vi "image calibrating and processing.vi"(3 "error in":errorcluster) -> (0 "error out":errorcluster, 1 "Objects Array":cluster{"X Coord":dbl[], "Y Coord":dbl[]}[](array[cluster]), 2 "Image Out (duplicate)":T1)   [LabVIEW 2009]
uses:
  <vilib>/vision/NI_Vision_Development_Module.lvlib
  <vilib>/vision/Image Controls.llb/IMAQ Image.ctl
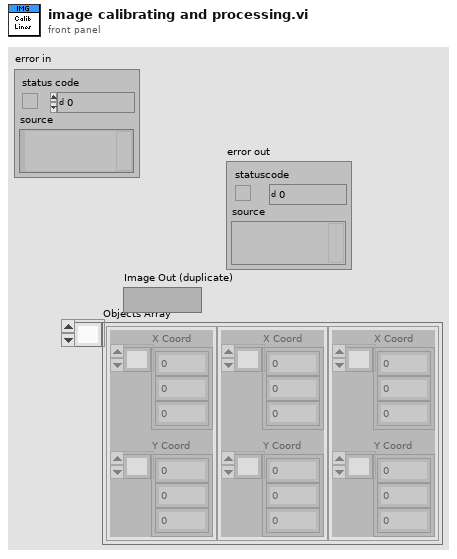
[diagram p1: front panel]
types:
  T1 = typedef "IMAQ Image.ctl" = refnum<image>
  T2 = enum32{"AutoM", "Close", "Dilate", "Erode", "Gradient", "Gradient out", "Gradient in", "Hit miss", "Open", "PClose", "POpen", "Thick", "Thin"}
  T3 = cluster{"Measurement Parameter":i32, "Range Lower Value":dbl, "Range Upper Value":dbl, "Range":bool, "Measurement Type":bool}[]
  T4 = typedef "Image Type" = u32
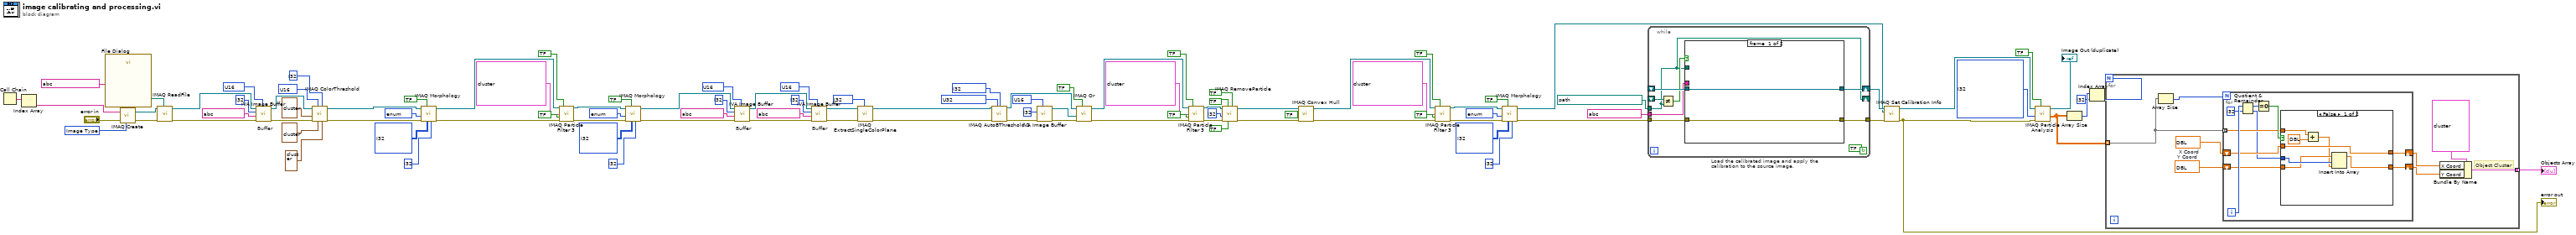
[diagram p0: block diagram]
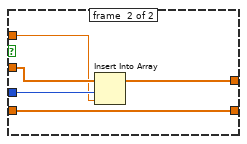
[diagram p2: hidden frame]
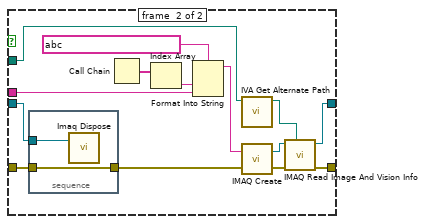
[diagram p3: hidden frame]
diagram:
  w10 = i32[] ? items=["Center of Mass X", "Center of Mass Y", "First Pixel X", "First Pixel Y", "Bounding Rect Left", "Bounding Rect Top", "Bounding Rect Right", "Bounding Rect Bottom", "Max Feret Diameter Start X", "Max Feret Diameter Start Y", "Max Feret Diameter End X", "Max Feret Diameter End Y", "Max Horiz. Segment Length Left", "Max Horiz. Segment Length Right", "Max Horiz. Segment Length Row", "-", "Bounding Rect Width", "Bounding Rect Height", "Bounding Rect Diagonal", "Perimeter", "Convex Hull Perimeter", "Holes' Perimeter", "Max Feret Diameter", "Equivalent Ellipse Major Axis", "Equivalent Ellipse Minor Axis", "Equivalent Ellipse Minor Axis (Feret)", "Equivalent Rect Long Side", "Equivalent Rect Short Side", "Equivalent Rect Diagonal", "Equivalent Rect Short Side (Feret)", "Average Horiz. Segment Length", "Average Vert. Segment Length", "Hydraulic Radius", "Waddel Disk Diameter", "-", "Area", "Holes' Area", "Particle & Holes' Area", "Convex Hull Area", "Image Area", "-", "Number of Holes", "Number of Horiz. Segments", "Number of Vert. Segments", "-", "Orientation", "Max Feret Diameter Orientation", "-", "% Area/Image Area", "% Area/(Particle & Holes' Area)", "Ratio of Equivalent Ellipse Axes", "Ratio of Equivalent Rect Sides", "-", "Elongation Factor", "Compactness Factor", "Heywood Circularity Factor", "Type Factor", "-", "Sum X", "Sum Y", "Sum XX", "Sum XY", "Sum YY", "Sum XXX", "Sum XXY", "Sum XYY", "Sum YYY", "-", "Moment of Inertia XX", "Moment of Inertia XY", "Moment of Inertia YY", "Moment of Inertia XXX", "Moment of Inertia XXY", "Moment of Inertia XYY", "Moment of Inertia YYY", "Norm. Moment of Inertia XX", "Norm. Moment of Inertia XY", "Norm. Moment of Inertia YY", "Norm. Moment of Inertia XXX", "Norm. Moment of Inertia XXY", "Norm. Moment of Inertia XYY", "Norm. Moment of Inertia YYY", "Hu Moment 1", "Hu Moment 2", "Hu Moment 3", "Hu Moment 4", "Hu Moment 5", "Hu Moment 6", "Hu Moment 7"] ("Real-World Measurements")
  w46 = u16 ? items=["Push", "Pop", "Reset"] ("Function")
  w48 = i32 ? items=["clustering", "entropy", "metric", "moments", "inter-class variance"] ("Method")
  w49 = u32 ? items=["Bright Objects", "Dark Objects"] ("Look For")
  w54 = i32 ? items=["Red", "Green", "Blue", "Hue", "Saturation", "Luminance", "Value", "Intensity"] ("Color Plane")
  w57 = u16 ? items=["Push", "Pop", "Reset"] ("Function")
  w62 = u16 ? items=["Push", "Pop", "Reset"] ("Function")
  w87 = u16 ? items=["RGB", "HSL", "HSV", "HSI"] ("Color Mode")
  w91 = u16 ? items=["Push", "Pop", "Reset"] ("Function")
  w94 = T4 ? items=["Grayscale (U8)", "Grayscale (I16)", "Grayscale (SGL)", "Complex (CSG)", "RGB (U32)", "HSL (U32)", "RGB (U64)", "Grayscale (U16)"] ("Image Type")
  # "Buffer"
  # "Buffer"
  # "Buffer"
  n1 = Call Chain() -> (call chain=w98:string[])
  n2 = Index Array(array=w98) -> (element=w97:string)  [unwired: 1 in]
  n3 = call "File Dialog"("prompt"=string ?) -> ("selected path"=w95:path)  [unwired: 6 in, 8 out]
  n4 = call "IMAQ Create"("Image Name"=w97, "Image Type"=w94, "error in (no error)"="error in") -> ("New Image"=w101:T1, "error out"=w100:errorcluster)  [unwired: 1 in, 1 out]
  n5 = call "IMAQ ReadFile"("File Path"=w95, "error in (no error)"=w100, "Image"=w101) -> ("error out"=w102:errorcluster, "Image Out"=w93:T1)  [unwired: 2 in, 5 out]
  n6 = call <vilib>:"IVA Image Buffer.vi"("Function"=w91, "error in (no error)"=w102, "Prefix"=string ?, "Buffer #"=i32 ?, "Image In"=w93) -> ("error out"=w92:errorcluster, "Image Out"=w83:T1)  [unwired: 5 out]
  n7 = call "IMAQ ColorThreshold"("Blue or Luma or Val or Inten Range"=cluster{"Lower value":i32, "Upper value":i32} ?, "Replace Value"=i32 ?, "Green or Sat Range"=cluster{"Lower value":i32, "Upper value":i32} ?, "Color Mode"=w87, "error in (no error)"=w92, "Red or Hue Range"=cluster{"Lower value":i32, "Upper value":i32} ?, "Image Src"=w83) -> ("error out"=w82:errorcluster, "Image Dst Out"=w77:T1)  [unwired: 1 in, 2 out]
  n8 = call "IMAQ Morphology"("Number of iterations (1)"=i32 ?, "Structuring Element"=i32[][] ?, "Square/Hexa (Square)"=bool ?, "error in (no error)"=w82, "Operation"=T2 ?, "Image Src"=w77) -> ("error out"=w76:errorcluster, "Image Dst Out"=w72:T1)  [unwired: 1 in, 3 out]
  n9 = call "IMAQ Particle Filter 3"("Image Src"=w72, "Connectivity 4/8 (8)"=bool ?, "Selection Values"=T3 ?, "Keep/Remove Particles (F)"=bool ? ("Keep/Remove Particles"), "error in (no error)"=w76) -> ("Image Dst Out"=w66:T1, "error out"=w73:errorcluster)  [unwired: 4 in, 5 out]
  n10 = call "IMAQ Morphology"("Number of iterations (1)"=i32 ?, "Structuring Element"=i32[][] ?, "Square/Hexa (Square)"=bool ?, "error in (no error)"=w73, "Operation"=T2 ?, "Image Src"=w66) -> ("error out"=w65:errorcluster, "Image Dst Out"=w64:T1)  [unwired: 1 in, 3 out]
  n11 = call <vilib>:"IVA Image Buffer.vi"("Function"=w62, "error in (no error)"=w65, "Prefix"=string ?, "Buffer #"=i32 ?, "Image In"=w64) -> ("error out"=w63:errorcluster, "Image Out"=w59:T1)  [unwired: 5 out]
  n12 = call <vilib>:"IVA Image Buffer.vi"("Function"=w57, "error in (no error)"=w63, "Prefix"=string ?, "Buffer #"=i32 ?, "Image In"=w59) -> ("error out"=w58:errorcluster, "Image Out"=w53:T1)  [unwired: 5 out]
  n13 = call "IMAQ ExtractSingleColorPlane"("Color Plane"=w54, "error in (no error)"=w58, "Image Src"=w53) -> ("error out"=w52:errorcluster, "Image Dst Out"=w51:T1)  [unwired: 1 in, 6 out]
  n14 = call "IMAQ AutoBThreshold 2"("Image Src"=w51, "Look For (Bright Objects)"=w49, "Method (clustering)"=w48, "error in (no error)"=w52) -> ("Image Dst Out"=w42:T1, "error out"=w50:errorcluster)  [unwired: 4 in, 6 out]
  n15 = call <vilib>:"IVA Image Buffer.vi"("Function"=w46, "error in (no error)"=w50, "Buffer #"=i32 ?) -> ("error out"=w43:errorcluster, "Image Out"=w44:T1)  [unwired: 2 in, 5 out]
  n16 = call "IMAQ Or"("Or/Nor (Or)"=bool ?, "error in (no error)"=w43, "Image Src B"=w44, "Image Src A"=w42) -> ("error out"=w41:errorcluster, "Image Dst Out"=w37:T1)  [unwired: 2 in, 4 out]
  n17 = call "IMAQ Particle Filter 3"("Image Src"=w37, "Connectivity 4/8 (8)"=bool ?, "Selection Values"=T3 ?, "Keep/Remove Particles (F)"=bool ? ("Keep/Remove Particles"), "error in (no error)"=w41) -> ("Image Dst Out"=w31:T1, "error out"=w38:errorcluster)  [unwired: 4 in, 5 out]
  n18 = call "IMAQ RemoveParticle"("Connectivity 4/8 (8)"=bool ?, "Low Pass/High Pass (Low)"=bool ?, "Square/Hexa (Square)"=bool ?, "error in (no error)"=w38, "Number of Erosion"=i32 ?, "Image Src"=w31) -> ("error out"=w30:errorcluster, "Image Dst Out"=w29:T1)  [unwired: 1 in, 3 out]
  n19 = call "IMAQ Convex Hull"("error in (no error)"=w30, "Connectivity 4/8 (8)"=bool ?, "Image Src"=w29) -> ("error out"=w27:errorcluster, "Image Dst Out"=w23:T1)  [unwired: 1 in, 6 out]
  n20 = call "IMAQ Particle Filter 3"("Image Src"=w23, "Connectivity 4/8 (8)"=bool ?, "Selection Values"=T3 ?, "Keep/Remove Particles (F)"=bool ? ("Keep/Remove Particles"), "error in (no error)"=w27) -> ("Image Dst Out"=w17:T1, "error out"=w24:errorcluster)  [unwired: 4 in, 5 out]
  n21 = call "IMAQ Morphology"("Number of iterations (1)"=i32 ?, "Structuring Element"=i32[][] ?, "Square/Hexa (Square)"=bool ?, "error in (no error)"=w24, "Operation"=T2 ?, "Image Src"=w17) -> ("error out"=w16:errorcluster, "Image Dst Out"=w12:T1)  [unwired: 1 in, 3 out]
  n22 = while "Load the calibrated image and apply the calibration to the source image." {
    shift-right: [w111] -> w14
    shift-left: _ -> [w110]
    tunnel: [w108] -> w13
    tunnel: w16 -> [w107]
    tunnel: path ? ("File Path") -> [w103]
    tunnel: string ? ("Step Name") -> [w106]
    shift-right: [w103] -> _
    shift-left: _ -> [w105]
    stop <- bool ? continue-if-true
    n23 = Not Equal?(x=w105, y=w103) -> (x != y?=w104:bool)
    n24 = case shown="True" w104 {
      tunnel: [w113 w125] -> w111
      tunnel: w110 -> [w113 w117]
      tunnel: [w112 w122] -> w108
      tunnel: w107 -> [w112 w118]
      tunnel: w103 -> [_ w115]
      tunnel: w106 -> [_ w119]
      frame #0 {
      }
      frame #1 {
        n25 = stacked-sequence {
          tunnel: w118 -> [w128]
          tunnel: w117 -> [w129]
          tunnel: [w128] -> w116
          frame #0 {
            n26 = call "Imaq Dispose"("Image"=w129) -> ()  [unwired: 2 in, 4 out]
          }
        }
        n27 = Call Chain() -> (call chain=w121:string[])
        n28 = Index Array(array=w121) -> (element=w120:string)  [unwired: 1 in]
        n29 = Format Into String(format string=string ? ("Image Name"), w120, w119) -> (resulting string=w127:string)  [unwired: 2 in, 1 out]
        n30 = call <vilib>:"IVA Get Alternate Path.vi"("Path In"=w115) -> ("Path Out"=w114:path)  [unwired: 10 out]
        n31 = call "IMAQ Create"("Image Name"=w127, "error in (no error)"=w116) -> ("New Image"=w124:T1, "error out"=w123:errorcluster)  [unwired: 2 in, 1 out]
        n32 = call "IMAQ Read Image And Vision Info"("File Path"=w114, "error in (no error)"=w123, "Image"=w124) -> ("error out"=w122:errorcluster, "Image Out"=w125:T1)  [unwired: 1 in, 6 out]
      }
    }
  }
  n33 = call "IMAQ Set Calibration Info"("error in (no error)"=w13, "Image Dst"=w12, "Image Src"=w14) -> ("error out"=w2:errorcluster, "Calibrated Image"=w9:T1)  [unwired: 1 in, 6 out]
  "error out" <- w2
  n34 = call "IMAQ Particle Analysis"("Connectivity 4/8 (8)"=bool ?, "error in (no error)"=w2, "Real-World Measurements"=w10, "Image"=w9) -> ("Particle Measurements (Real-World)"=w4:dbl[][], "Image Out (duplicate)"=→"Image Out (duplicate)":T1)  [unwired: 1 in, 5 out]
  n35 = Array Size(array=w4) -> (size(s)=w7:i32[])
  n36 = Index Array(array=w7, index=i32 ?) -> (element=w5:i32)
  n37 = for {
    N: w5 -> [_]
    tunnel: w4 -> [w134] mode=indexing
    tunnel: [w130] -> w3 mode=indexing
    w135 = dbl[] ?  # Y Coord
    w136 = dbl[] ?  # X Coord
    # "Object Cluster"
    n38 = Array Size(array=w134) -> (size(s)=w137:i32)
    n39 = for {
      N: w137 -> [_]
      tunnel: w134 -> [w141] mode=indexing
      shift-right: [w139] -> w132
      shift-left: w136 -> [w143]
      shift-right: [w138] -> w131
      shift-left: w135 -> [w142]
      i -> [w147]
      n40 = Quotient & Remainder(x=w147, y=i32 ?) -> (x-y*floor(x/y)=w145:i32, floor(x/y)=w140:i32)
      n41 = Equal To 0?(x=w145) -> (x = 0?=w144:bool)
      n42 = case shown="False" w144 {
        tunnel: w143 -> [w153 w159]
        tunnel: w142 -> [w152 w155]
        tunnel: w141 -> [w149 w156]
        tunnel: w140 -> [w154 w158]
        tunnel: [w153 w157] -> w139
        tunnel: [w151 w155] -> w138
        frame #0 {
          n43 = Add(x=w149, y=dbl ?) -> (x+y=w148:dbl)
          n44 = Insert Into Array(array=w152, index=w154, new element=w148) -> (w151:dbl[])
        }
        frame #1 {
          n45 = Insert Into Array(array=w159, index=w158, new element=w156) -> (w157:dbl[])
        }
      }
    }
    n46 = Bundle By Name(cluster=cluster{"X Coord":dbl[], "Y Coord":dbl[]} ?, "X Coord"=w132, "Y Coord"=w131) -> (w130:cluster{"X Coord":dbl[], "Y Coord":dbl[]})
  }
  "Objects Array" <- w3
